vi "SMO.UI.Example.TestLauncher.vi"() -> ()   [LabVIEW 2013, in "SMO.UI.Example.lvclass"]
uses:
  SMO.UI.Example.lvclass
  SMO/Typedefs/SMOState --Enum.ctl
  SMO/SMO.lvclass
  SMO.UI/SMO.UI.lvclass
panel:
  out "error out":errorcluster
  in  "Stop":bool
  # "SMO.UI Test Launcher"
  # "For instructions on how to use the JKI State Machine Objects, examples and video tutorials, visit:\nhttp://jki.net/state-machine-objects/\n\nJKI State Machine Objects™\nhttp://jki.net/state-machine-objects/\nCopyright (C) 2005-2015, JKI <info@jki.net>\nALL RIGHTS RESERVED"
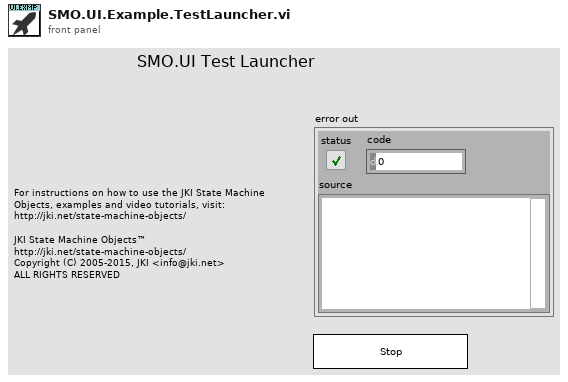
[diagram p1: front panel]
types:
  T1 = typedef "SMO.lvclass/Public Events.ctl" = cluster{"Error":refnum<user-event>, "State":refnum<user-event>}
  T2 = typedef "SMO.UI.lvclass/PublicEvents--Cluster.ctl" = cluster{"UI Hidden":refnum<user-event>, "UI State":refnum<user-event>}
  T3 = typedef "SMO.lvclass/SMOState --Enum.ctl" = enum16{"unknown", "Created", "Started", "Stopped"}
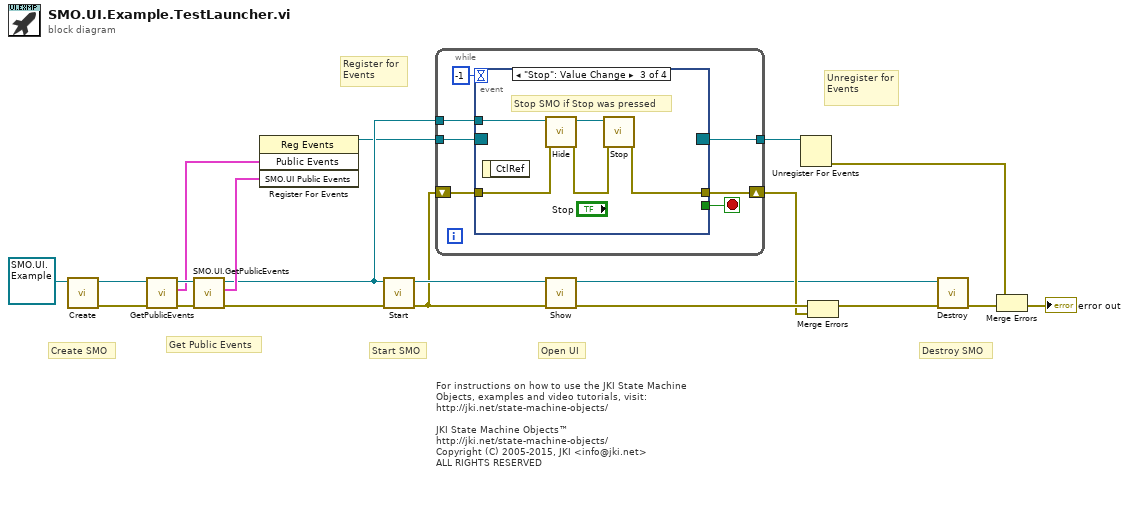
[diagram p0: block diagram]
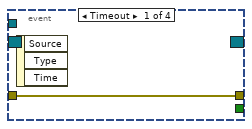
[diagram p2: hidden frame]
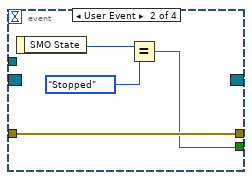
[diagram p3: hidden frame]
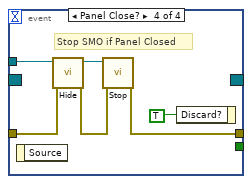
[diagram p4: hidden frame]
diagram:
  # "For instructions on how to use the JKI State Machine Objects, examples and video tutorials, visit:\nhttp://jki.net/state-machine-objects/\n\nJKI State Machine Objects™\nhttp://jki.net/state-machine-objects/\nCopyright (C) 2005-2015, JKI <info@jki.net>\nALL RIGHTS RESERVED"
  # "Get Public Events"
  # "Start SMO"
  # "Destroy SMO"
  # "Create SMO"
  # "Open UI"
  # "Unregister for Events"
  # "Register for Events"
  n1 = call "Create.vi"("SMO"=refnum<class "SMO.UI.Example.lvclass"> refnum ("SMO.UI.Example.lvclass")) -> ("error out"=w5:errorcluster, "SMO out"=w7:refnum<class "SMO.UI.Example.lvclass">)  [unwired: 8 in, 1 out]
  n2 = call "GetPublicEvents.vi"("error in (no error)"=w5, "SMO"=w7) -> ("error out"=w10:errorcluster, "Public Events"=w8:T1, "SMO out"=w9:refnum<class "SMO.UI.Example.lvclass">)  [unwired: 7 in]
  n3 = call "SMO.UI.GetPublicEvents.vi"("error in (no error)"=w10, "SMO.UI"=w9) -> ("error out"=w4:errorcluster, "SMO.UI Public Events"=w11:T2, "SMO.UI out"=w6:refnum<class "SMO.UI.Example.lvclass">)  [unwired: 7 in]
  n4 = register-events(w8, w11) -> (reference out=w3:refnum<event-registration>)  [unwired: 2 in, 1 out]
  n5 = call "Start.vi"("error in (no error)"=w4, "SMO"=w6) -> ("error out"=w17:errorcluster, "SMO out"=w19:refnum<class "SMO.UI.Example.lvclass">)  [unwired: 8 in]
  n6 = while {
    shift-right: [w26] -> w16
    shift-left: w17 -> [w25]
    tunnel: w3 -> [w24]
    tunnel: [w23] -> w20
    tunnel: w6 -> [w22]
    stop <- w27 stop-if-true
    n7 = event shown="[2] \"Stop\": Value Change" {
      selector: w24 -> [_ _ _ _]
      dyn-events: [_ _ _ _] -> w23
      timeout: -1 -> [_ _ _ _]
      tunnel: [_ w29 _ _] -> w27
      tunnel: w22 -> [_ _ w36 w41]
      tunnel: [w28 w32 w37 w43] -> w26
      tunnel: w25 -> [w28 w32 w34 w39]
      event Timeout {
        n8 = event-data() -> ()  [unwired: 1 in, 3 out]
      }
      event User Event {
        n9 = event-data() -> ("SMO State"=w31:T3)  [unwired: 1 in]
        n10 = Equal?(x=w31, y=SMOState_--Enum."Stopped") -> (x = y?=w29:bool)
      }
      event "Stop": Value Change {
        # "Stop SMO if Stop was pressed"
        n11 = event-data() -> ()  [unwired: 1 in, 1 out]
        n12 = call "Hide.vi"("error in (no error)"=w34, "SMO.UI"=w36) -> ("error out"=w33:errorcluster, "SMO.UI out"=w35:refnum<class "SMO.UI.Example.lvclass">)  [unwired: 8 in]
        n13 = call "Stop.vi"("error in (no error)"=w33, "SMO"=w35) -> ("error out"=w37:errorcluster)  [unwired: 8 in, 1 out]
      }
      event Panel Close? {
        # "Stop SMO if Panel Closed"
        n14 = event-data() -> ()  [unwired: 1 in, 1 out]
        n15 = call "Hide.vi"("error in (no error)"=w39, "SMO.UI"=w41) -> ("error out"=w38:errorcluster, "SMO.UI out"=w40:refnum<class "SMO.UI.Example.lvclass">)  [unwired: 8 in]
        n16 = call "Stop.vi"("error in (no error)"=w38, "SMO"=w40) -> ("error out"=w43:errorcluster)  [unwired: 8 in, 1 out]
        n17 = event-data("Discard?"=TRUE ("OK")) -> ()  [unwired: 1 in, 1 out]
      }
    }
  }
  n18 = call "Show.vi"("error in (no error)"=w17, "SMO.UI"=w19) -> ("error out"=w18:errorcluster, "SMO.UI out"=w2:refnum<class "SMO.UI.Example.lvclass">)  [unwired: 8 in]
  n19 = Unregister For Events(event registration refnum=w20) -> (error out=w15:errorcluster)  [unwired: 1 in]
  n20 = Merge Errors(w18, w16) -> (w1:errorcluster)
  n21 = call "Destroy.vi"("error in (no error)"=w1, "SMO"=w2) -> ("error out"=w12:errorcluster)  [unwired: 9 in]
  n22 = Merge Errors(w15, w12) -> (→"error out":errorcluster)
